vi "STAGE+mono+counter_edit9.vi"() -> ()   [LabVIEW 2017]
uses:
  Control 1.ctl
panel:
  out "Slide":u8(slide) max=10 step=10 scale=0.0..10.0
  out "XY Graph":cluster{dbl[], dbl[]}(graph)
  out "Waveform Graph 2":waveform(dbl)(graph) caption="Record 41  of  100"
  in  "?":enum32{"DELAY", "COUNTER", "MONO"}(tab)
  out "Final time [ps]":dbl
  out "Current time [ps]":dbl
  out "Initial time [ps]":dbl
  in  "Set this as t0":bool
  in  "Axis":i32=1
  in  "Motor ON":bool
  in  "Motor OFF":bool
  out "Current Position [mm]":dbl
  out "Final Position [mm]":dbl
  in  "Data Points":i32=100
  out "Current Point":i32
  in  "Step Size [um]":i32=10
  in  "Averaging Time [s]":dbl=0.1
  in  "Rep Rate [Hz]":dbl=500.0
  out "Shots":dbl
  in  "Target [mm]":dbl format="%.3f"
  in  "Move":bool
  out "Initial position [mm]":dbl
  in  "GPIB address":string="23"
  in  "Count Mode":u16(ring) items=["A,B for Preset T", "A-B for Preset T", "A+B for Preset T", "A for Preset B"]
  in  "Trigger mode":u16(ring) items=["10 MHz"=0, "Input 2"=2, "Input T"=3]
  in  "Channel A Input":u16(ring)=1 items=["10 MHz", "Input 1"]
  in  "Channel B Input":u16(ring)=2 items=["Input 1"=1, "Input 2"=2]
  in  "Number of Measurements\n to take at one point/ Number of Periods":u16=1 min=1 max=2000 step=1
  in  "Time between measurements\n at one point (s)/Dwell Time":dbl=0.002 min=0.002 max=60.0 step=0.001
  in  "gate A mode (CW:0)":i16(slide) scale=0.0..2.0 scale format="%.2f"
  out "Counts":i32
  in  "Integrating time, 10^-7 sec":dbl=10000000.0
  out "Mono port":T1(ring)
  out "Time delay":u32=450000 min=1
  out "Serial":u32=12345
  in  "Step size":dbl=10.0 min=0.0
  in  "Scan to":i32=4000
  in  "Scan from":i32=2600
  out "Current wavelength":dbl
  out "Grt#":u8=1 min=1 max=3 step=1
  in  "?":bool
  out "Groove/mm":u32=1200
  out "Blaze (nm)":u32=300
  out "Timeout 2":bool
  in  "?":bool
  out "Timeout":bool
  in  "Collect Data!":bool
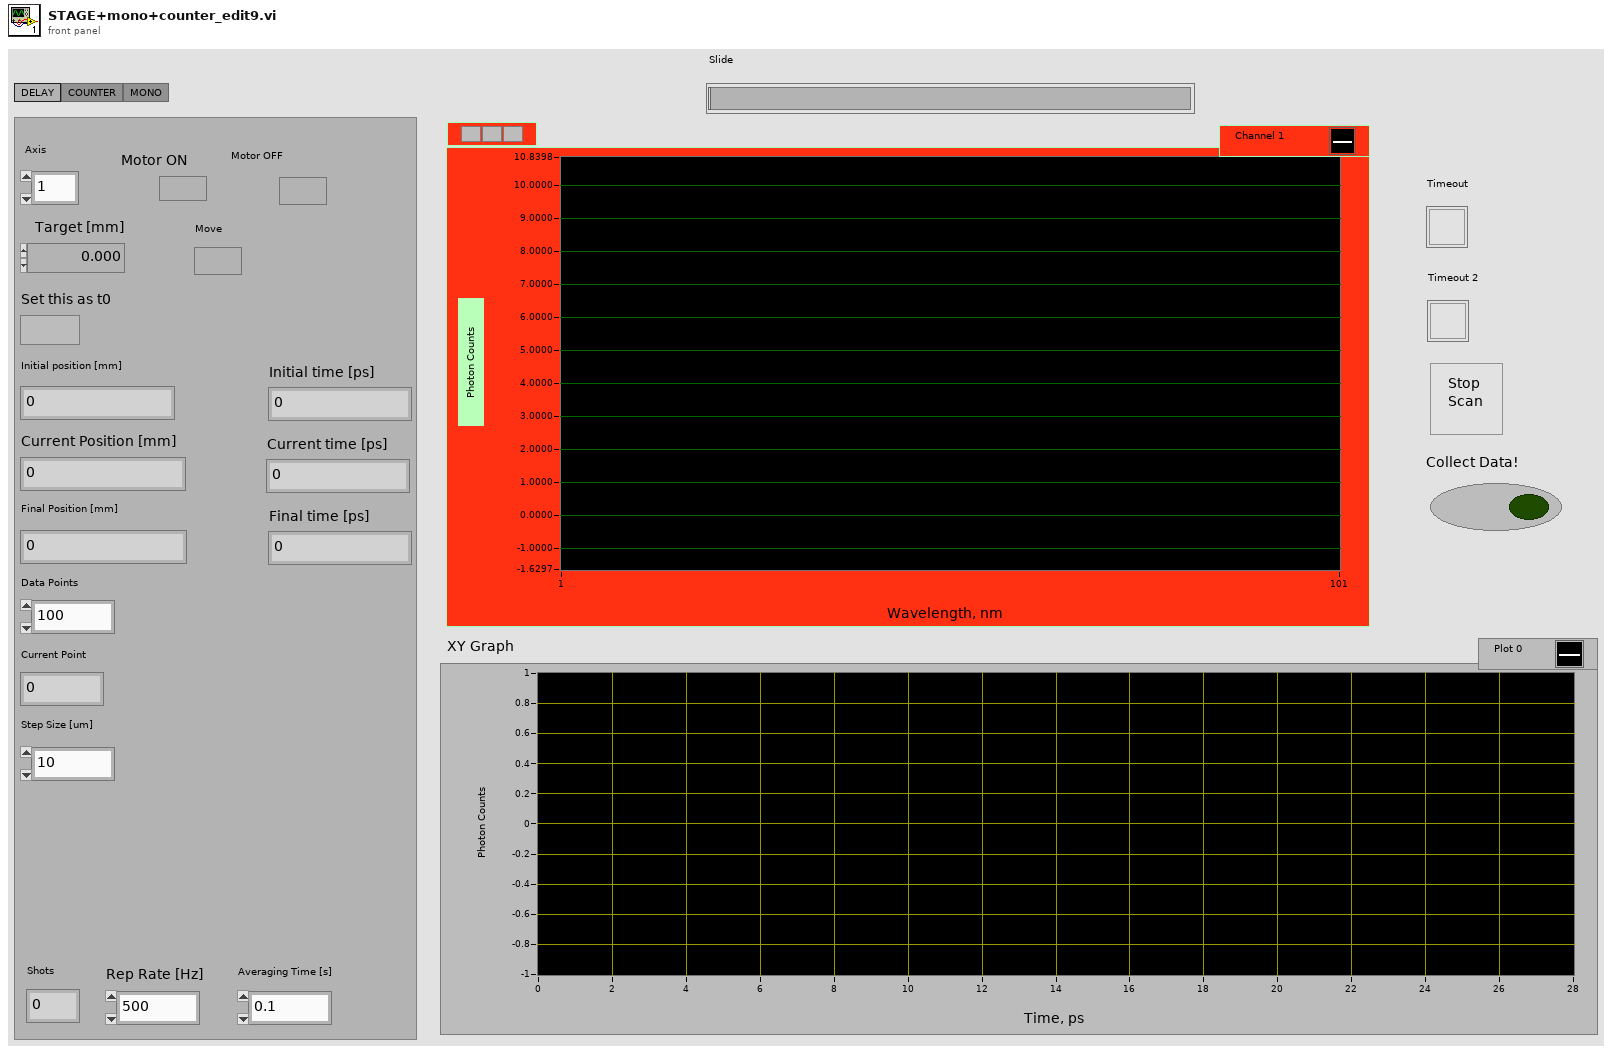
[diagram p1: front panel]
types:
  T1 = enum8{"COM 1", "COM 2", "COM 3", "COM 4", "COM 5", "COM 6", "COM 7", "COM 8", "COM 9"}
  T2 = cluster{"input XON/XOFF":bool, "input HW Handshake":bool, "input alt HW HShk":bool, "output XON/XOFF":bool, "output HW Handshake":bool, "output alt HW HShk":bool, "XOFF byte":u8, "XON byte":u8, "parity error byte":u16}
  T3 = enum16{"no parity", "odd parity", "even parity", "mark parity", "space parity"}
  T4 = typedef "Control 1.ctl" = dbl[]
  T5 = cluster{"Y[0]":dbl, "Y[1]":dbl, "Y[2]":dbl, "Y[3]":dbl, "Y[4]":dbl, "Y[5]":dbl, "Y[6]":dbl, "Y[7]":dbl, "Y[8]":dbl}
  T6 = typedef "NI_Matrix.lvlib/RealMatrix.ctl" = dbl[][]
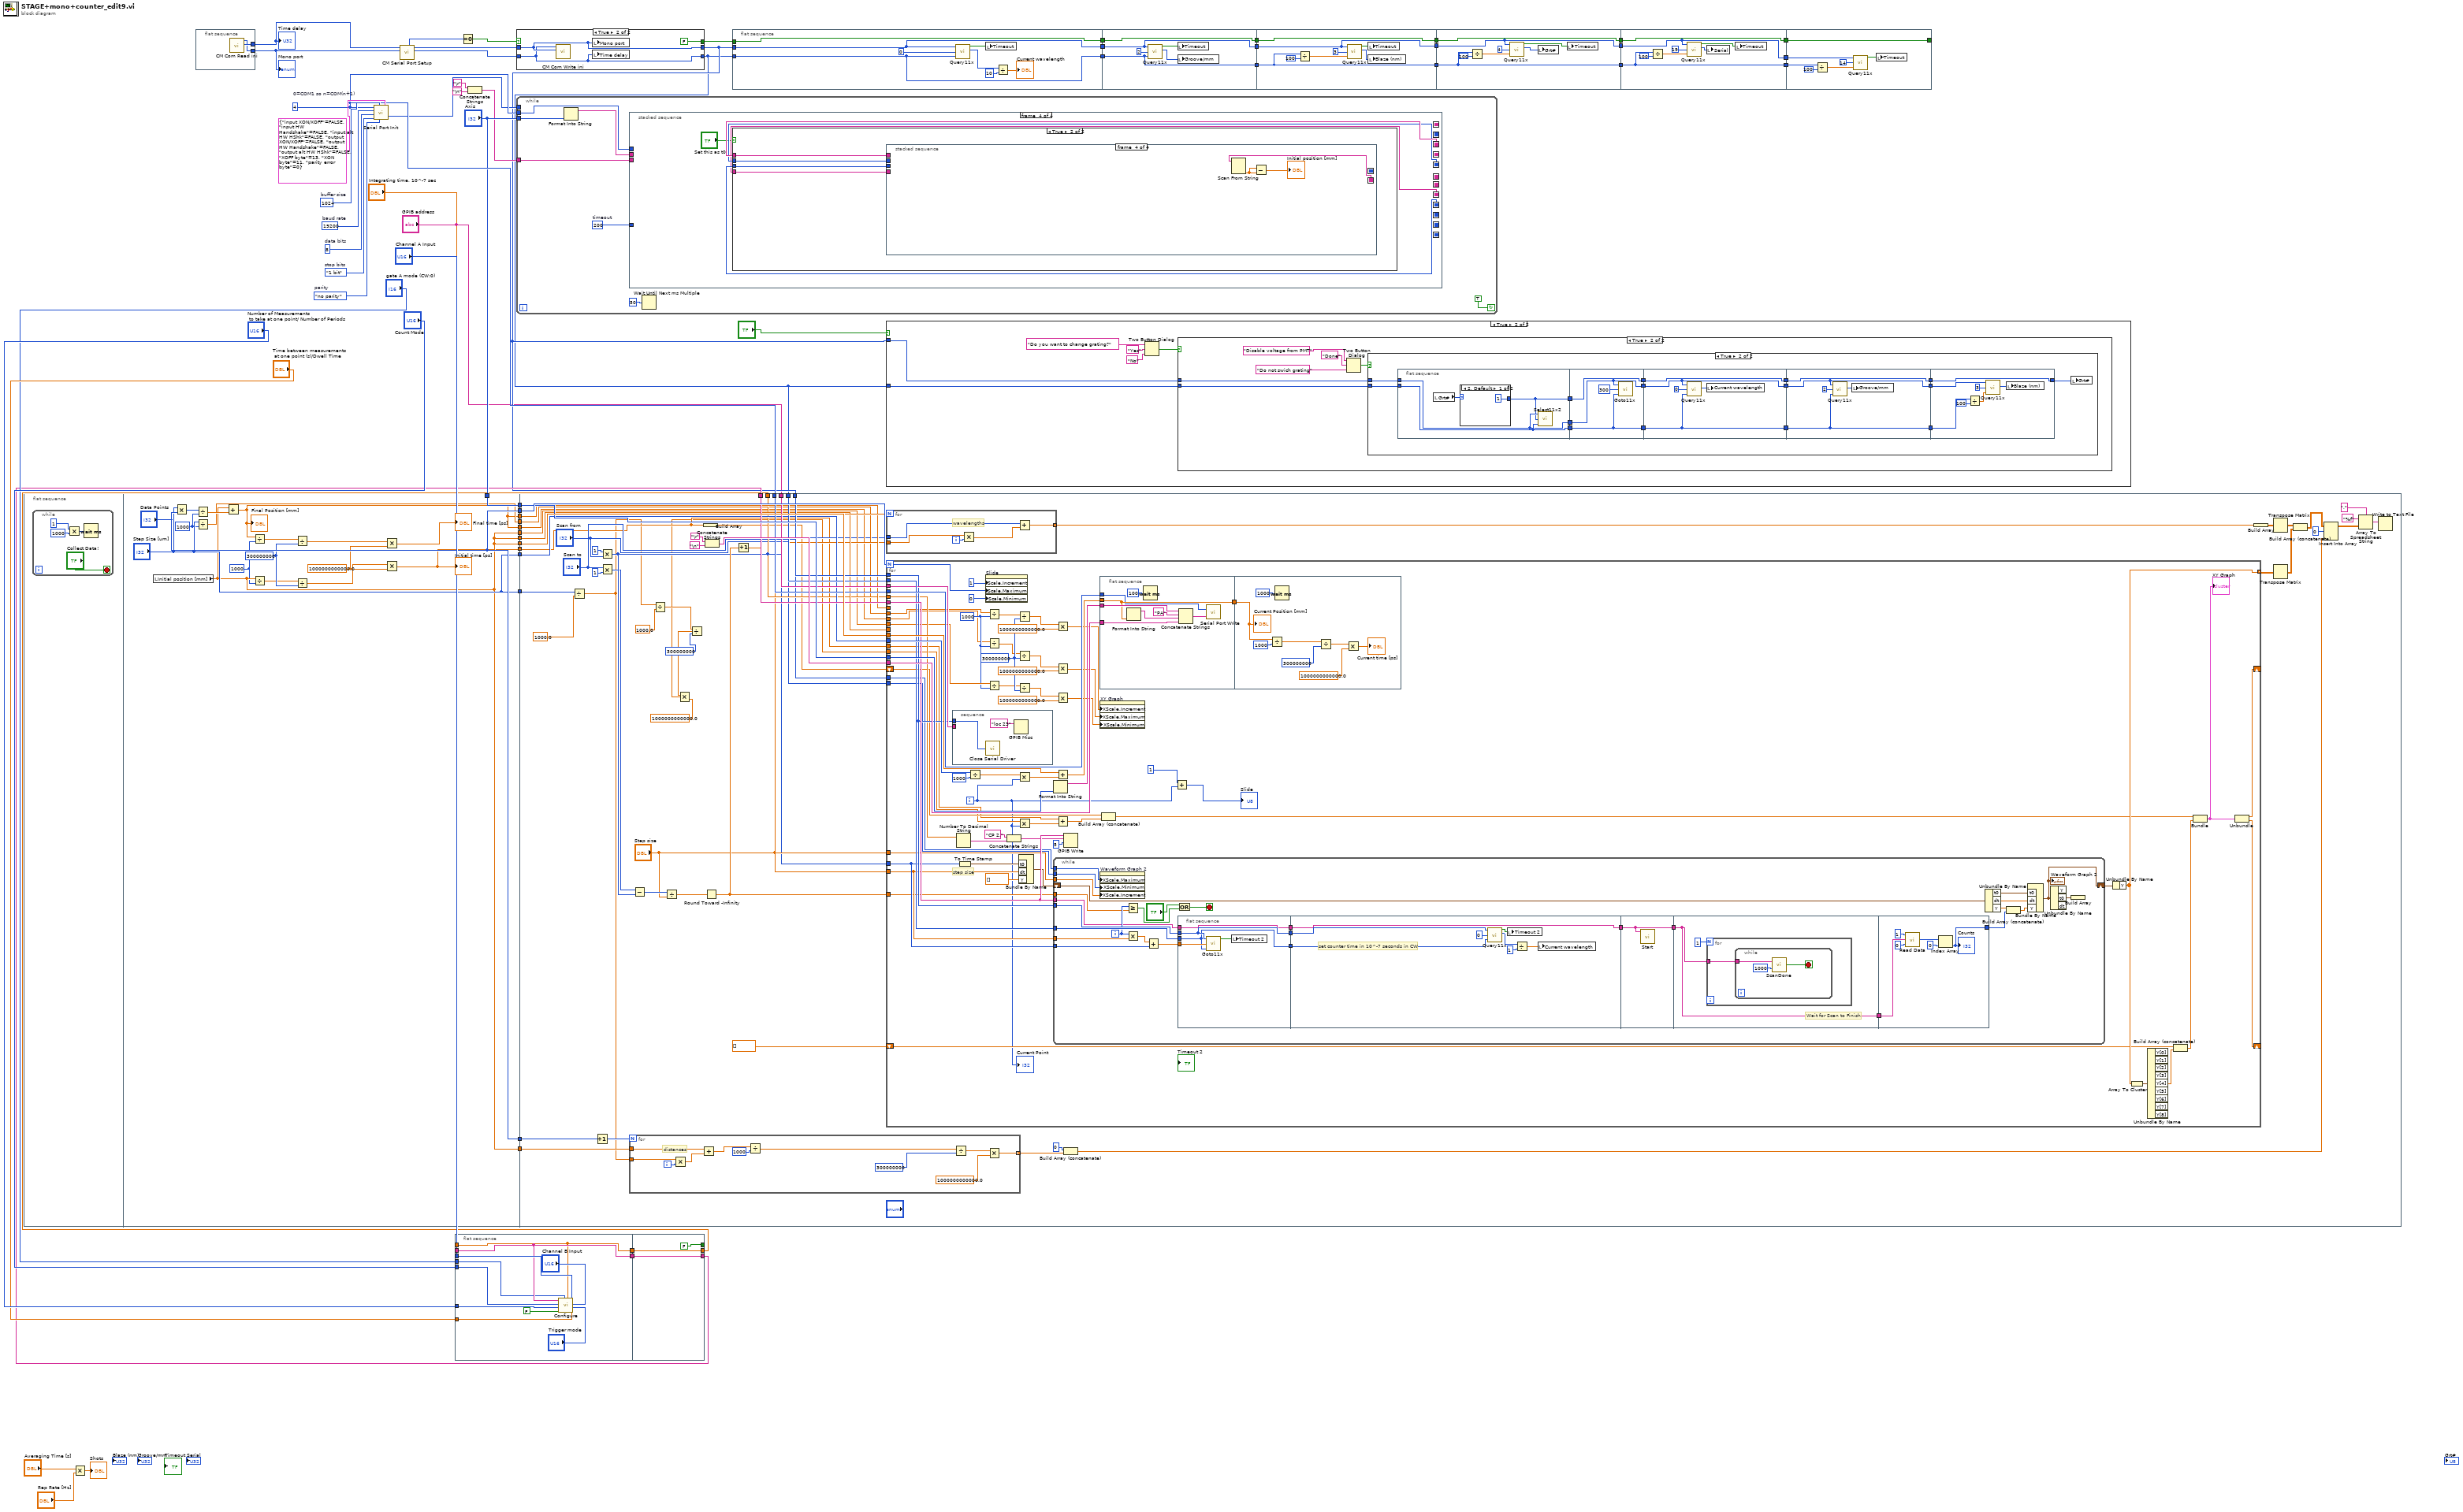
[diagram p0: block diagram]
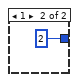
[diagram p5: hidden frame]
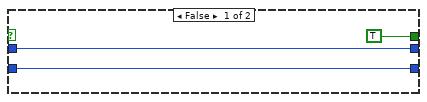
[diagram p6: hidden frame]
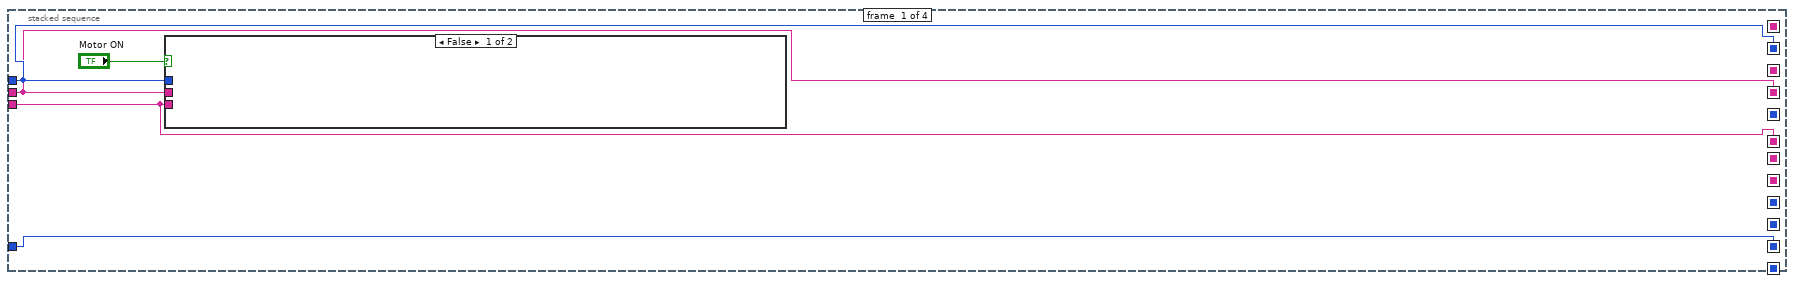
[diagram p7: hidden frame]
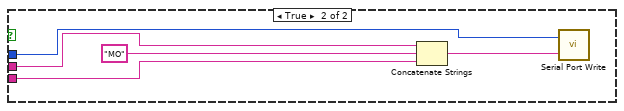
[diagram p8: hidden frame]
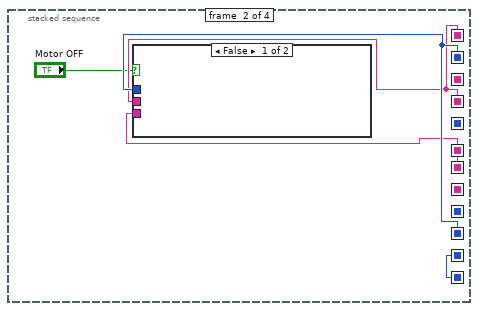
[diagram p9: hidden frame]
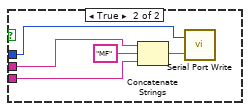
[diagram p10: hidden frame]
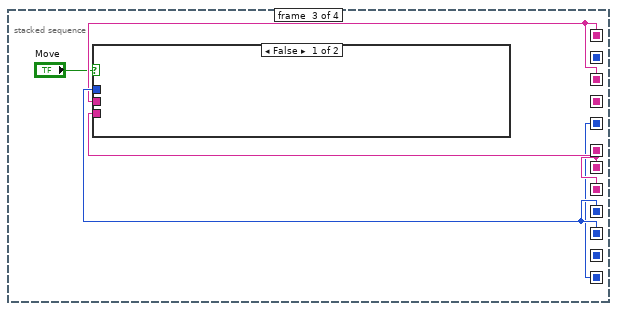
[diagram p11: hidden frame]
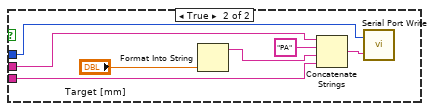
[diagram p12: hidden frame]
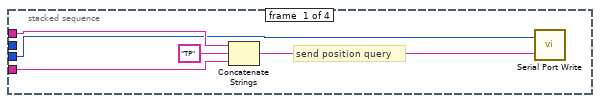
[diagram p14: hidden frame]
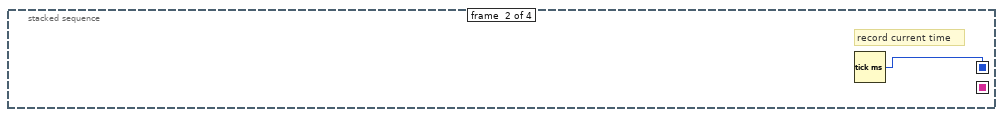
[diagram p15: hidden frame]
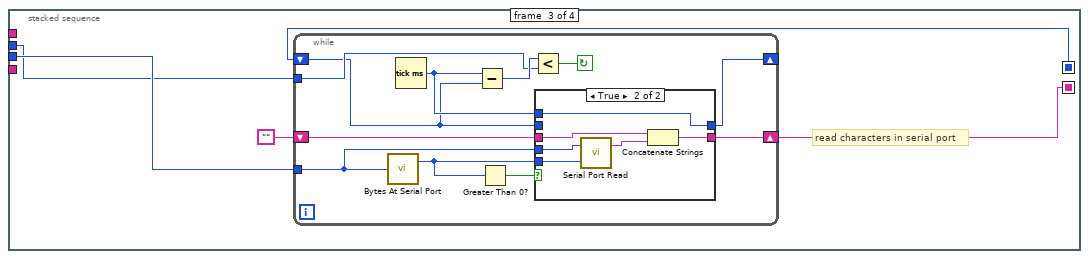
[diagram p16: hidden frame]
diagram:
  w55 = u32 19200  # baud rate
  w54 = u16 8  # data bits
  w53 = enum16{"1 bit", "1.5 bits", "2 bits"}."1 bit"  # stop bits
  w58 = T3."no parity"  # parity
  w52 = 4  # 0=COM1 so n=COM(n+1)
  w57 = u16 1024  # buffer size
  n1 = flat-sequence {
    tunnel: ["Data Points"] -> w64
    tunnel: "Axis" -> [w86]
    tunnel: [w78] -> w63
    tunnel: [w86] -> w62
    tunnel: ["Step Size [um]"] -> w12
    tunnel: [w78] -> w11
    tunnel: ["Step Size [um]"] -> w10
    tunnel: ["Data Points"] -> w9
    tunnel: [w78] -> w8
    tunnel: [w77] -> w7
    tunnel: [w78] -> w4
    tunnel: [w77] -> w3
    tunnel: [w80] -> w2
    tunnel: [w69] -> w1
    tunnel: w64 -> [w144]
    tunnel: w63 -> [w143]
    tunnel: w62 -> [w142]
    tunnel: w52 -> [w138]
    tunnel: w16 -> [w137]
    tunnel: w15 -> [w136]
    tunnel: w14 -> [w135]
    tunnel: "GPIB address" -> [w134]
    tunnel: w12 -> [w119]
    tunnel: w11 -> [w117]
    tunnel: w10 -> [w116]
    tunnel: w9 -> [w114]
    tunnel: w8 -> [w107]
    tunnel: w7 -> [w106]
    tunnel: w6 -> [w105]
    tunnel: w4 -> [w101]
    tunnel: w3 -> [w100]
    tunnel: w2 -> [w99]
    tunnel: w1 -> [w94]
    frame #0 {
      n2 = while {
        stop <- "Collect Data!" stop-if-true
        n3 = Multiply(x=1, y=1000) -> (x*y=w68:i32)
        n4 = Wait (ms)(milliseconds to wait=w68) -> ()  [unwired: 1 out]
      }
    }
    frame #1 {
      w70 = 1000000000000.0
      w76 = 1000
      w79 = 300000000
      w81 = 1000
      n5 = local read "Initial position [mm]"() -> (w78:dbl)
      n6 = Multiply(x="Step Size [um]", y="Data Points") -> (x*y=w85:i32)
      n7 = Divide(x=w85, y=w81) -> (x/y=w84:dbl)
      n8 = Divide(x="Step Size [um]", y=w81) -> (x/y=w80:dbl)
      n9 = Add(x=w78, y=w84) -> (x+y=w77:dbl)
      "Final Position [mm]" <- w77
      n10 = Divide(x=w77, y=w76) -> (x/y=w75:dbl)
      n11 = Divide(x=w78, y=w76) -> (x/y=w74:dbl)
      n12 = Divide(x=w75, y=w79) -> (x/y=w72:dbl)
      n13 = Divide(x=w74, y=w79) -> (x/y=w73:dbl)
      n14 = Multiply(x=w72, y=w70) -> (x*y=→"Final time [ps]":dbl)
      n15 = Multiply(x=w73, y=w70) -> (x*y=w69:dbl)
      "Initial time [ps]" <- w69
    }
    frame #2 {
      n16 = Divide(x=w119, y=1000.0) -> (x/y=w88:dbl)
      n17 = Increment(x=w114) -> (x+1=w115:i32)
      n18 = Multiply(x=1, y="Scan from") -> (x*y=w96:i32)
      n19 = Multiply(x="Scan to", y=1) -> (x*y=w95:i32)
      n20 = for {
        N: w115 -> [_]
        tunnel: w88 -> [w155]
        tunnel: w117 -> [w153]
        tunnel: [w146] -> w113 mode=indexing
        i -> [w154]
        # "distances"
        n21 = Multiply(x=w155, y=w154) -> (x*y=w152:dbl)
        n22 = Add(x=w153, y=w152) -> (x+y=w151:dbl)
        n23 = Divide(x=w151, y=1000) -> (x/y=w145:dbl)
        n24 = Divide(x=w145, y=300000000) -> (x/y=w148:dbl)
        n25 = Multiply(x=w148, y=1000000000000.0) -> (x*y=w146:dbl)
      }
      n26 = Subtract(x=w95, y=w96) -> (x-y=w129:i32)
      n27 = Divide(x=w88, y=1000.0) -> (x/y=w89:dbl)
      n28 = Divide(x=w129, y="Step size") -> (x/y=w128:dbl)
      n29 = Divide(x=w89, y=300000000) -> (x/y=w91:dbl)
      n30 = Multiply(x=w91, y=1000000000000.0) -> (x*y=w87:dbl)
      n31 = Build Array(w94) -> (w97:dbl[])
      n32 = Round Toward -Infinity(1:w128) -> (0:w127:dbl)
      n33 = Concatenate Strings("\r", "\n") -> (w139:string)
      n34 = Increment(x=w127) -> (x+1=w126:dbl)
      n35 = for {
        N: w126 -> [_]
        tunnel: "Step size" -> [w160]
        tunnel: w96 -> [w158]
        tunnel: [w156] -> w124 mode=indexing
        i -> [w159]
        # "wavelengths"
        n36 = Multiply(x=w160, y=w159) -> (x*y=w157:dbl)
        n37 = Add(x=w158, y=w157) -> (x+y=w156:dbl)
      }
      n38 = for {
        N: w144 -> [w184]
        tunnel: w143 -> [w227]
        tunnel: w116 -> [w223]
        tunnel: w142 -> [w220]
        tunnel: w139 -> [w217]
        tunnel: w138 -> [w218]
        tunnel: w137 -> [w216]
        tunnel: w136 -> [w213]
        tunnel: w135 -> [w215]
        tunnel: w134 -> [w214]
        tunnel: [w201] -> w122 mode=indexing
        tunnel: w96 -> [w204]
        tunnel: "Step size" -> [w203]
        tunnel: w127 -> [w202]
        tunnel: w107 -> [_]
        tunnel: w106 -> [_]
        tunnel: w105 -> [w199]
        tunnel: "Scan to" -> [w198]
        tunnel: "Scan from" -> [w197]
        tunnel: "Step size" -> [w196]
        tunnel: w101 -> [w179]
        tunnel: w100 -> [w177]
        tunnel: w99 -> [w180]
        tunnel: w87 -> [w164]
        shift-right: [w194] -> _
        shift-left: w97 -> [w189]
        shift-right: [w191] -> _
        shift-left: T4 [] ("Y") -> [w190]
        tunnel: w94 -> [w188]
        i -> [w163]
        w178 = 1000
        w181 = 300000000
        # "step size"
        n39 = stacked-sequence {
          tunnel: w213 -> [w284]
          tunnel: w214 -> [_]
          frame #0 {
            n40 = call <vilib>:"Close Serial Driver.vi"("port number"=w284) -> ()  [unwired: 1 out]
            n41 = GPIB Misc(0:"loc 23" ("command string")) -> ()  [unwired: 1 in, 3 out]
          }
        }
        n42 = Number To Decimal String(number=w199) -> (decimal integer string=w208:string)  [unwired: 1 in]
        n43 = To Time Stamp(1:w204) -> (0:w211:timestamp)
        n44 = Divide(x=w223, y=1000) -> (x/y=w222:dbl)
        n45 = property on="Slide" class="Slide (strict)"("Scale.Increment"=1, "Scale.Maximum"=w184, "Scale.Minimum"=0) -> ()  [unwired: 2 in, 2 out]
        n46 = Divide(x=w180, y=w178) -> (x/y=w176:dbl)
        n47 = Divide(x=w177, y=w178) -> (x/y=w174:dbl)
        n48 = Divide(x=w179, y=w178) -> (x/y=w175:dbl)
        n49 = Concatenate Strings("CP 2,", w208) -> (w206:string)
        n50 = Divide(x=w176, y=w181) -> (x/y=w170:dbl)
        n51 = Divide(x=w174, y=w181) -> (x/y=w166:dbl)
        n52 = Divide(x=w175, y=w181) -> (x/y=w168:dbl)
        n53 = Multiply(x=w222, y=w163) -> (x*y=w226:dbl)
        n54 = Multiply(x=w164, y=w163) -> (x*y=w195:dbl)
        n55 = Bundle By Name("t0"=w211, "dt"=w203, "Y"=dbl[] []) -> (w210:waveform(dbl))  [unwired: 1 in]
        n56 = Format Into String(w220) -> (resulting string=w219:string)  [unwired: 3 in, 1 out]
        n57 = while {
          tunnel: w213 -> [w255]
          tunnel: w215 -> [w254]
          shift-right: [w229] -> w205
          shift-left: w210 -> [w252]
          tunnel: w216 -> [w244]
          tunnel: w204 -> [w235]
          tunnel: w203 -> [w234]
          tunnel: w202 -> [w233]
          tunnel: w198 -> [w232]
          tunnel: w197 -> [w231]
          tunnel: w196 -> [w230]
          i -> [w249]
          stop <- w253 stop-if-true
          n58 = property on="Waveform Graph 2" class="WFGraph (strict)"("XScale.Maximum"=w232, "XScale.Minimum"=w231, "XScale.Increment"=w230) -> ()  [unwired: 2 in, 2 out]
          n59 = Greater Or Equal?(x=w249, y=w233) -> (x >= y?=w245:bool)
          n60 = Multiply(x=w249, y=w234) -> (x*y=w256:dbl)
          n61 = Add(x=w256, y=w235) -> (x+y=w236:dbl)
          n62 = Or(x="?", y=w245) -> (x .or. y?=w253:bool)
          n63 = flat-sequence {
            tunnel: w236 -> [w261]
            tunnel: w255 -> [w260]
            tunnel: [w260] -> w242
            tunnel: w254 -> [w259]
            tunnel: [w259] -> w241
            tunnel: w244 -> [w257]
            tunnel: [w257] -> w240
            tunnel: w242 -> [w268]
            tunnel: w241 -> [w267]
            tunnel: w240 -> [w265]
            tunnel: [w265] -> w239
            tunnel: w239 -> [w270]
            tunnel: [w270] -> w238
            tunnel: w238 -> [w271]
            tunnel: [w271] -> w237
            tunnel: w237 -> [w278]
            tunnel: [w277] -> w243
            frame #0 {
              n64 = call "Goto11x.vi"("time delay"=w259, "WAVELENGTH"=w261, "port number"=w260) -> ("timeout"=w258:bool)  [unwired: 2 out]
              n65 = local write "Timeout 2"(w258) -> ()
            }
            frame #1 {
              # "set counter time in 10^-7 seconds in CW"
              n66 = call "Query11x.vi"("port number"=w268, "QUERY"=0, "time delay"=w267) -> ("timeout"=w266:bool, "STATUS MESSAGE"=w264:u16)  [unwired: 2 out]
              n67 = local write "Timeout 2"(w266) -> ()
              n68 = Divide(x=w264, y=1) -> (x/y=w263:dbl)
              n69 = local write "Current wavelength"(w263) -> ()
            }
            frame #2 {
              n70 = call "Start.vi"("GPIB Address"=w270) -> ()  [unwired: 9 in]
            }
            frame #3 {
              # "Wait for Scan to Finish"
              n71 = for {
                N: 1 -> [_]
                tunnel: w271 -> [w273]
                n72 = while {
                  tunnel: w273 -> [w274]
                  stop <- w276 stop-if-true
                  n73 = call "ScanDone.vi"("Wait (ms)"=1000, "GPIB Address"=w274) -> ("Scan Finished?"=w276:bool)
                }
              }
            }
            frame #4 {
              n74 = call "Read Data.vi"("Channel Number"=0, "GPIB Address"=w278, "Number of Datapoints"=1) -> ("Data"=w279:i32[])
              n75 = Index Array(array=w279, index=0) -> (element=w277:i32)
              "Counts" <- w277
            }
          }
          n76 = Unbundle By Name(w252) -> ("t0"=w250:timestamp, "dt"=w251:dbl, "Y"=w248:dbl[])
          n77 = Build Array (concatenate)(w248, w243) -> (w247:dbl[])
          n78 = Bundle By Name("t0"=w250, "dt"=w251, "Y"=w247) -> (w229:waveform(dbl))  [unwired: 1 in]
          "Waveform Graph 2" <- w229
          n79 = Unbundle By Name(w229) -> ("t0"=w228:timestamp)  [unwired: 2 out]
          n80 = Build Array(w228) -> ()  [unwired: 1 out]
        }
        n81 = Multiply(x=w170, y=1000000000000.0) -> (x*y=w169:dbl)
        n82 = Multiply(x=w166, y=1000000000000.0) -> (x*y=w165:dbl)
        n83 = Multiply(x=w168, y=1000000000000.0) -> (x*y=w167:dbl)
        n84 = Add(x=w227, y=w226) -> (x+y=w225:dbl)
        n85 = Add(x=w188, y=w195) -> (x+y=w187:dbl)
        n86 = GPIB Write(0:w216, 1:w206, 2:i16 5 ("mode (0)")) -> ()  [unwired: 2 in, 2 out]
        n87 = flat-sequence {
          tunnel: w225 -> [w287]
          tunnel: [w287] -> w221
          tunnel: w217 -> [w289]
          tunnel: w219 -> [w288]
          tunnel: w218 -> [w285]
          tunnel: w221 -> [w298]
          frame #0 {
            n88 = Format Into String(w287) -> (resulting string=w286:string)  [unwired: 3 in, 1 out]
            n89 = Wait (ms)(milliseconds to wait=u32 100) -> ()  [unwired: 1 out]
            n90 = Concatenate Strings(w288, "PA" ("Substring"), w286, w289) -> (w291:string)
            n91 = call <vilib>:"Serial Port Write.vi"("string to write"=w291, "port number"=w285) -> ()  [unwired: 1 out]
          }
          frame #1 {
            n92 = Divide(x=w298, y=1000) -> (x/y=w296:dbl)
            n93 = Wait (ms)(milliseconds to wait=u32 1000) -> ()  [unwired: 1 out]
            n94 = Divide(x=w296, y=300000000) -> (x/y=w295:dbl)
            n95 = Multiply(x=w295, y=1000000000000.0) -> (x*y=→"Current time [ps]":dbl)
            "Current Position [mm]" <- w298
          }
        }
        n96 = property on="XY Graph" class="XYGraph (strict)"("XScale.Increment"=w169, "XScale.Maximum"=w165, "XScale.Minimum"=w167) -> ()  [unwired: 2 in, 2 out]
        n97 = Build Array (concatenate)(w189, w187) -> (w186:dbl[])
        n98 = Add(x=1, y=w163) -> (x+y=→"Slide":i32)
        n99 = Unbundle By Name(w205) -> ("Y"=w201:dbl[])
        n100 = Array To Cluster(array=w201) -> (cluster=w200:T5)
        n101 = Unbundle By Name(w200) -> ("Y[4]"=w193:dbl)  [unwired: 8 out]
        n102 = Build Array (concatenate)(w190, w193) -> (w192:T4)
        n103 = Bundle(w186, "Y"=w192) -> (w185:cluster{dbl[], "Y":T4})  [unwired: 1 in]
        "XY Graph" <- w185
        n104 = Unbundle(w185) -> (w194:dbl[], "Y"=w191:T4)
        "Current Point" <- w163
      }
      n105 = Build Array (concatenate)(0, w113) -> (w110:dbl[])
      n106 = Build Array(w124) -> (w123:dbl[][])
      n107 = Transpose Matrix(1:w123) -> (0:w121:dbl[][])
      n108 = Transpose Matrix(1:w122) -> (0:w120:dbl[][])
      n109 = Build Array (concatenate)(w121, w120) -> (w109:T6)
      n110 = Insert Into Array(array=w109, index (row)=0, new element=w110) -> (w108:T6)  [unwired: 1 in]
      n111 = Array To Spreadsheet String(delimiter (Tab)=",", array=w108, 3:"%f" ("format string")) -> (spreadsheet string=w125:string)
      n112 = Write to Text File(text=w125) -> ()  [unwired: 3 in, 3 out]
    }
  }
  n113 = Multiply(x="Averaging Time [s]", y="Rep Rate [Hz]") -> (x*y=→"Shots":dbl)
  n114 = flat-sequence {
    tunnel: [w302] -> w30
    tunnel: [w301] -> w29
    frame #0 {
      n115 = call "CM Com Read ini.vi"() -> ("Mono port"=w301:T1, "time delay1"=w302:u32)  [unwired: 7 in]
    }
  }
  n116 = call <vilib>:"Serial Port Init.vi"("flow control etc."=T2 {"input XON/XOFF"=FALSE, "input HW Handshake"=FALSE, "input alt HW HShk"=FALSE, "output XON/XOFF"=FALSE, "output HW Handshake"=FALSE, "output alt HW HShk"=FALSE, "XOFF byte"=13, "XON byte"=11, "parity error byte"=0}, "parity"=w58, "buffer size"=w57, "stop bits"=w53, "data bits"=w54, "baud rate"=w55, "port number"=w52) -> ("error code"=w51:i32)
  n117 = call "CM Serial Port Setup.vi"("COM port"=w29, "time delay"=w30) -> ("time delay1"=w25:u32, "DK port Out"=w26:T1, "error code"=w28:i32)  [unwired: 7 in]
  n118 = flat-sequence {
    tunnel: "GPIB address" -> [w310]
    tunnel: [w310] -> w31
    tunnel: "Count Mode" -> [w311]
    tunnel: "Number of Measurements\n to take at one point/ Number of Periods" -> [w308]
    tunnel: "Time between measurements\n at one point (s)/Dwell Time" -> [w307]
    tunnel: "Channel A Input" -> [w312]
    tunnel: "gate A mode (CW:0)" -> [w304]
    tunnel: "Integrating time, 10^-7 sec" -> [w303]
    tunnel: [w303] -> w5
    tunnel: w31 -> [w314]
    tunnel: [w314] -> w16
    tunnel: [FALSE] -> _
    tunnel: [w313] -> w6
    tunnel: w5 -> [w313]
    frame #0 {
      n119 = call "Configure.vi"("Dwell Time (s)"=w307, "Channel T Input"="Trigger mode", "Channel B Input"="Channel B Input", "Channel A Input"=w312, "Integrating time, 10^-7 sec"=w303, "gate mode (CW:0)"=w304, "Scan End Mode"=FALSE, "Number of Periods"=w308, "Count Mode"=w311, "GPIB Address"=w310) -> ()
    }
    frame #1 {
    }
  }
  n120 = Equal To 0?(x=w28) -> (x = 0?=w27:bool)
  n121 = Concatenate Strings("\r", "\n") -> (w47:string)
  n122 = case shown="True" w27 {
    tunnel: w26 -> [w318 w321]
    tunnel: w25 -> [w317 w320]
    tunnel: [w318 w321] -> w15
    tunnel: [w317 w320] -> w14
    tunnel: [TRUE FALSE] -> w24
    frame False {
    }
    frame True {
      n123 = call "CM Com Write ini.vi"("time delay1"=w321, "Mono port"=w320) -> ()  [unwired: 7 in]
      n124 = local write "Mono port"(w321) -> ()
      n125 = local write "Time delay"(w320) -> ()
    }
  }
  n126 = while {
    tunnel: w52 -> [w324]
    tunnel: w47 -> [w325]
    tunnel: w51 -> [_]
    tunnel: "Axis" -> [w322]
    stop <- TRUE continue-if-true
    w323 = u32 200  # timeout
    n127 = Format Into String(w322) -> (resulting string=w326:string)  [unwired: 3 in, 1 out]
    n128 = stacked-sequence {
      seq-local: [w331 _ _ _] -> [_ w342 _ _]
      seq-local: [w330 _ _ _] -> [_ w341 _ _]
      seq-local: [w332 _ _ _] -> [_ w343 _ _]
      seq-local: [w329 _ _ _] -> [_ w339 _ _]
      seq-local: [_ w342 _ _] -> [_ _ w352 _]
      seq-local: [_ w341 _ _] -> [_ _ w351 _]
      seq-local: [_ w343 _ _] -> [_ _ w353 _]
      seq-local: [_ w339 _ _] -> [_ _ w349 _]
      seq-local: [_ _ w352 _] -> [_ _ _ w365]
      seq-local: [_ _ w351 _] -> [_ _ _ w362]
      seq-local: [_ _ w353 _] -> [_ _ _ w364]
      seq-local: [_ _ w349 _] -> [_ _ _ w363]
      tunnel: w326 -> [w331 _ _ _]
      tunnel: w325 -> [w330 _ _ _]
      tunnel: w324 -> [w332 _ _ _]
      tunnel: w323 -> [w329 _ _ _]
      frame #0 {
        n129 = case shown="False" "Motor ON" {
          tunnel: w332 -> [_ w338]
          tunnel: w331 -> [_ w335]
          tunnel: w330 -> [_ w334]
          frame False {
          }
          frame True {
            n130 = Concatenate Strings(w335, "MO" ("Substring"), w334) -> (w336:string)
            n131 = call <vilib>:"Serial Port Write.vi"("string to write"=w336, "port number"=w338) -> ()  [unwired: 1 out]
          }
        }
      }
      frame #1 {
        n132 = case shown="False" "Motor OFF" {
          tunnel: w343 -> [_ w348]
          tunnel: w342 -> [_ w345]
          tunnel: w341 -> [_ w344]
          frame False {
          }
          frame True {
            n133 = Concatenate Strings(w345, "MF" ("Substring"), w344) -> (w346:string)
            n134 = call <vilib>:"Serial Port Write.vi"("string to write"=w346, "port number"=w348) -> ()  [unwired: 1 out]
          }
        }
      }
      frame #2 {
        n135 = case shown="False" "Move" {
          tunnel: w353 -> [_ w360]
          tunnel: w352 -> [_ w357]
          tunnel: w351 -> [_ w356]
          frame False {
          }
          frame True {
            n136 = Format Into String("Target [mm]") -> (resulting string=w354:string)  [unwired: 3 in, 1 out]
            n137 = Concatenate Strings(w357, "PA" ("Substring"), w354, w356) -> (w358:string)
            n138 = call <vilib>:"Serial Port Write.vi"("string to write"=w358, "port number"=w360) -> ()  [unwired: 1 out]
          }
        }
      }
      frame #3 {
        n139 = case shown="True" "Set this as t0" {
          tunnel: w365 -> [_ w369]
          tunnel: w364 -> [_ w368]
          tunnel: w363 -> [_ w367]
          tunnel: w362 -> [_ w366]
          frame False {
          }
          frame True {
            n140 = stacked-sequence {
              seq-local: [_ w375 _ _] -> [_ _ w377 _]
              seq-local: [_ _ w376 _] -> [_ _ _ w402]
              tunnel: w369 -> [w372 _ _ _]
              tunnel: w368 -> [w371 _ w380 _]
              tunnel: w367 -> [_ _ w378 _]
              tunnel: w366 -> [w370 _ _ _]
              frame #0 {
                # "send position query"
                n141 = Concatenate Strings(w372, "TP" ("Substring"), w370) -> (w373:string)
                n142 = call <vilib>:"Serial Port Write.vi"("string to write"=w373, "port number"=w371) -> ()  [unwired: 1 out]
              }
              frame #1 {
                # "record current time"
                n143 = Tick Count (ms)() -> (millisecond timer value=w375:u32)
              }
              frame #2 {
                # "read characters in serial port"
                n144 = while {
                  shift-left: w377 -> [w381]
                  shift-right: [w382] -> _
                  tunnel: w378 -> [w385]
                  shift-left: "" -> [w388]
                  shift-right: [w387] -> w376
                  tunnel: w380 -> [w389]
                  stop <- w384 continue-if-true
                  n145 = call <vilib>:"Bytes At Serial Port.vi"("port number"=w389) -> ("byte count"=w390:u32)  [unwired: 1 out]
                  n146 = Tick Count (ms)() -> (millisecond timer value=w383:u32)
                  n147 = Subtract(x=w383, y=w381) -> (x-y=w386:u32)
                  n148 = Greater Than 0?(x=w390) -> (x > 0?=w391:bool)
                  n149 = Less?(x=w386, y=w385) -> (x < y?=w384:bool)
                  n150 = case shown="True" w391 {
                    tunnel: w390 -> [_ w399]
                    tunnel: w389 -> [_ w398]
                    tunnel: w388 -> [w393 w396]
                    tunnel: [w393 w395] -> w387
                    tunnel: [w392 w394] -> w382
                    tunnel: w383 -> [_ w394]
                    tunnel: w381 -> [w392 _]
                    frame False {
                    }
                    frame True {
                      n151 = call <vilib>:"Serial Port Read.vi"("requested byte count"=w399, "port number"=w398) -> ("string read"=w397:string)  [unwired: 1 out]
                      n152 = Concatenate Strings(w396, w397) -> (w395:string)
                    }
                  }
                }
              }
              frame #3 {
                n153 = Scan From String(input string=w402) -> (output 1=w400:dbl)  [unwired: 4 in, 3 out]
                n154 = Subtract(x=w400, y=w400) -> (x-y=→"Initial position [mm]":dbl)
              }
            }
          }
        }
      }
    }
    n155 = Wait Until Next ms Multiple(millisecond multiple=u32 50) -> ()  [unwired: 1 out]
  }
  n156 = flat-sequence {
    tunnel: w14 -> [w408]
    tunnel: [w408] -> w46
    tunnel: w15 -> [w410]
    tunnel: [w410] -> w45
    tunnel: w24 -> [w406]
    tunnel: [w406] -> w44
    tunnel: w46 -> [w413]
    tunnel: [w413] -> w43
    tunnel: w45 -> [w415]
    tunnel: [w415] -> w42
    tunnel: w44 -> [w411]
    tunnel: [w411] -> w41
    tunnel: w43 -> [w423]
    tunnel: [w423] -> w40
    tunnel: w42 -> [w420]
    tunnel: [w420] -> w39
    tunnel: w41 -> [w417]
    tunnel: [w417] -> w38
    tunnel: w40 -> [w431]
    tunnel: [w431] -> w37
    tunnel: w39 -> [w428]
    tunnel: [w428] -> w36
    tunnel: w38 -> [w425]
    tunnel: [w425] -> w35
    tunnel: w37 -> [w439]
    tunnel: [w439] -> w34
    tunnel: w36 -> [w436]
    tunnel: [w436] -> w33
    tunnel: w35 -> [w433]
    tunnel: [w433] -> w32
    tunnel: w34 -> [w446]
    tunnel: w33 -> [w443]
    tunnel: [w441] -> _
    tunnel: w32 -> [w441]
    frame #0 {
      n157 = call "Query11x.vi"("port number"=w410, "QUERY"=u16 0, "time delay"=w408) -> ("timeout"=w407:bool, "STATUS MESSAGE"=w405:u16)  [unwired: 2 out]
      n158 = local write "Timeout"(w407) -> ()
      n159 = Divide(x=w405, y=10 ("Numeric")) -> (x/y=→"Current wavelength":dbl)
    }
    frame #1 {
      n160 = call "Query11x.vi"("port number"=w415, "QUERY"=u16 2, "time delay"=w413) -> ("timeout"=w412:bool, "STATUS MESSAGE"=w414:u16)  [unwired: 2 out]
      n161 = local write "Timeout"(w412) -> ()
      n162 = local write "Groove/mm"(w414) -> ()
    }
    frame #2 {
      n163 = Divide(x=w423, y=i16 100 ("device (1)")) -> (x/y=w421:dbl)
      n164 = call "Query11x.vi"("port number"=w420, "QUERY"=u16 3, "time delay"=w421) -> ("timeout"=w418:bool, "STATUS MESSAGE"=w419:u16)  [unwired: 2 out]
      n165 = local write "Timeout"(w418) -> ()
      n166 = local write "Blaze (nm)"(w419) -> ()
    }
    frame #3 {
      n167 = Divide(x=w431, y=i16 100 ("device (1)")) -> (x/y=w429:dbl)
      n168 = call "Query11x.vi"("port number"=w428, "QUERY"=u16 4, "time delay"=w429) -> ("timeout"=w426:bool, "STATUS MESSAGE"=w427:u16)  [unwired: 2 out]
      n169 = local write "Grt#"(w427) -> ()
      n170 = local write "Timeout"(w426) -> ()
    }
    frame #4 {
      n171 = Divide(x=w439, y=i16 100 ("device (1)")) -> (x/y=w437:dbl)
      n172 = call "Query11x.vi"("port number"=w436, "QUERY"=u16 19, "time delay"=w437) -> ("timeout"=w434:bool, "STATUS MESSAGE"=w435:u16)  [unwired: 2 out]
      n173 = local write "Serial"(w435) -> ()
      n174 = local write "Timeout"(w434) -> ()
    }
    frame #5 {
      n175 = Divide(x=w446, y=i16 100 ("device (1)")) -> (x/y=w444:dbl)
      n176 = call "Query11x.vi"("port number"=w443, "QUERY"=u16 14, "time delay"=w444) -> ("timeout"=w442:bool)  [unwired: 3 out]
      n177 = local write "Timeout"(w442) -> ()
    }
  }
  n178 = case shown="True" "?" {
    tunnel: w14 -> [_ w449]
    tunnel: w15 -> [_ w448]
    frame False {
    }
    frame True {
      n179 = Two Button Dialog(message="Do you want to change grating?", 1:"No" ("F button name (\"Cancel\")"), 2:"Yes" ("T button name (\"OK\")")) -> (T button?=w450:bool)
      n180 = case shown="True" w450 {
        tunnel: w449 -> [_ w455]
        tunnel: w448 -> [_ w454]
        frame False {
        }
        frame True {
          n181 = Two Button Dialog(message="Disable voltage from PMT", 1:"Do not swich grating" ("F button name (\"Cancel\")"), 2:"Done" ("T button name (\"OK\")")) -> (T button?=w456:bool)
          n182 = case shown="True" w456 {
            tunnel: w455 -> [_ w474]
            tunnel: w454 -> [_ w473]
            frame False {
            }
            frame True {
              n183 = flat-sequence {
                tunnel: w474 -> [w478]
                tunnel: [w478] -> w471
                tunnel: w473 -> [w477]
                tunnel: [w477] -> w470
                tunnel: [w475] -> w469
                tunnel: w471 -> [w482]
                tunnel: [w482] -> w468
                tunnel: w470 -> [w483]
                tunnel: [w483] -> w467
                tunnel: w469 -> [w481]
                tunnel: [w481] -> w466
                tunnel: w468 -> [w489]
                tunnel: [w489] -> w465
                tunnel: w467 -> [w488]
                tunnel: [w488] -> w464
                tunnel: w466 -> [w486]
                tunnel: [w486] -> w463
                tunnel: w465 -> [w492]
                tunnel: [w492] -> w462
                tunnel: w464 -> [w493]
                tunnel: [w493] -> w461
                tunnel: w463 -> [w490]
                tunnel: [w490] -> w460
                tunnel: w462 -> [w497]
                tunnel: w461 -> [w498]
                tunnel: [w495] -> w472
                tunnel: w460 -> [w495]
                frame #0 {
                  n184 = local read "Grt#"() -> (w476:u8)
                  n185 = case shown="2, Default" w476 {
                    tunnel: [1 2] -> w475
                    frame 2, Default {
                    }
                    frame 1 {
                    }
                  }
                  n186 = call "Select11x2.vi"("time delay"=w478, "NEW GRT?"=w475, "port number"=w477) -> ()  [unwired: 3 out]
                }
                frame #1 {
                  n187 = call "Goto11x.vi"("time delay"=w482, "WAVELENGTH"=u16 300, "port number"=w483) -> ()  [unwired: 3 out]
                }
                frame #2 {
                  n188 = call "Query11x.vi"("port number"=w488, "QUERY"=u16 0, "time delay"=w489) -> ("STATUS MESSAGE"=w485:u16)  [unwired: 3 out]
                  n189 = local write "Current wavelength"(w485) -> ()
                }
                frame #3 {
                  n190 = call "Query11x.vi"("port number"=w493, "QUERY"=u16 2, "time delay"=w492) -> ("STATUS MESSAGE"=w491:u16)  [unwired: 3 out]
                  n191 = local write "Groove/mm"(w491) -> ()
                }
                frame #4 {
                  n192 = Divide(x=w497, y=i16 100 ("device (1)")) -> (x/y=w499:dbl)
                  n193 = call "Query11x.vi"("port number"=w498, "QUERY"=u16 3, "time delay"=w499) -> ("STATUS MESSAGE"=w496:u16)  [unwired: 3 out]
                  n194 = local write "Blaze (nm)"(w496) -> ()
                }
              }
              n195 = local write "Grt#"(w472) -> ()
            }
          }
        }
      }
    }
  }
  "Mono port" <- w29
  "Time delay" <- w30
